vi "PegaRetaOrientacaoOuPosicaovi.vi"(4 "Goal Width":u32, 5 "Field Length":u32, 6 "Orientação inimigo":dbl format="%#_13g", 7 "Meio?":bool=TRUE, 8 "Y bola":dbl format="%#_13g", 9 "X bola":dbl format="%#_13g", 10 "Y inimigo":dbl format="%#_13g", 11 "X inimigo":dbl format="%#_13g") -> (0 "Orientação goleiro":dbl format="%#_13g", 2 "Y goleiro":dbl format="%#_13g", 3 "X goleiro":dbl format="%#_13g")   [LabVIEW 2017]
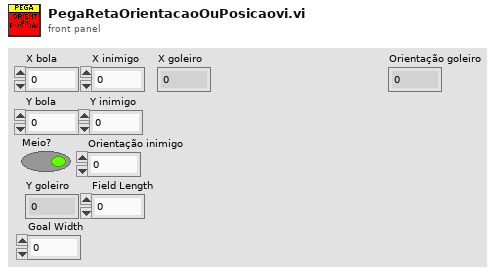
[diagram p1: front panel]
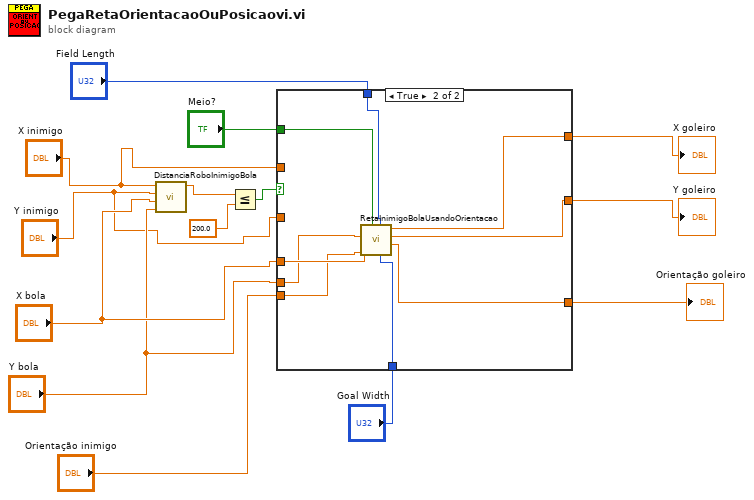
[diagram p0: block diagram]
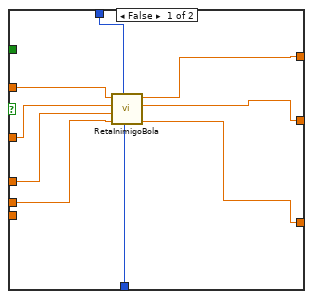
[diagram p2: hidden frame]
diagram:
  n1 = call "DistanciaRoboInimigoBola.vi"("Y bola"="Y bola", "X bola"="X bola", "Y inimigo"="Y inimigo", "X inimigo"="X inimigo") -> ("Distância"=w14:dbl)  [unwired: 5 in, 2 out]
  n2 = Less Or Equal?(x=w14, y=200.0) -> (x <= y?=w12:bool)
  n3 = case shown="True" w12 {
    tunnel: "X bola" -> [w23 w32]
    tunnel: "Y bola" -> [w22 w31]
    tunnel: "Orientação inimigo" -> [_ w30]
    tunnel: "Meio?" -> [_ w29]
    tunnel: "Goal Width" -> [w18 w28]
    tunnel: "Field Length" -> [w19 w27]
    tunnel: [w17 w26] -> w5
    tunnel: [w16 w25] -> w4
    tunnel: [w15 w24] -> w3
    tunnel: "X inimigo" -> [w21 _]
    tunnel: "Y inimigo" -> [w20 _]
    frame False {
      n4 = call "RetaInimigoBola.vi"("Goal width"=w18, "Field lenght"=w19, "Y bola"=w22, "X bola"=w23, "Y inimigo"=w20, "X inimigo"=w21) -> ("Orientação"=w15:dbl, "Y goleiro"=w16:dbl, "X goleiro"=w17:dbl)  [unwired: 3 in]
    }
    frame True {
      n5 = call "RetaInimigoBolaUsandoOrientacao.vi"("Goal Width"=w28, "Field length"=w27, "Meio?"=w29, "Orientação inimigo"=w30, "Y bola"=w31, "X bola"=w32) -> ("Orientação goleiro"=w24:dbl, "Y golerio"=w25:dbl, "X goleiro"=w26:dbl)  [unwired: 3 in]
    }
  }
  "X goleiro" <- w5
  "Y goleiro" <- w4
  "Orientação goleiro" <- w3
